vi "Hswitch.vi"(8 "Joy val":dbl, 10 "High Limit Switch":bool) -> (3 "LiftVal":dbl)   [LabVIEW 2017]
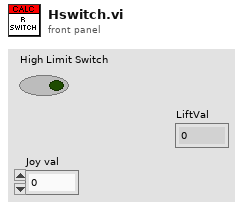
[diagram p1: front panel]
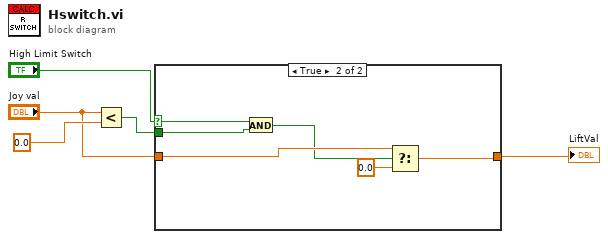
[diagram p0: block diagram]
diagram:
  n1 = Less?(x="Joy val", y=0.0) -> (x < y?=w1:bool)
  n2 = case shown="True" "High Limit Switch" {
    selector: "High Limit Switch" -> [_ w8]
    tunnel: "Joy val" -> [w6 w12]
    tunnel: [w6 w11] -> w3
    tunnel: w1 -> [_ w7]
    frame False {
    }
    frame True {
      n3 = And(x=w8, y=w7) -> (x .and. y?=w9:bool)
      n4 = Select(t=w12, s=w9, f=0.0) -> (s? t:f=w11:dbl)
    }
  }
  "LiftVal" <- w3
